vi "ALTS-2015 Display Sensor ID.vi"(8 "error in (no error)":errorcluster) -> (0 "error out":errorcluster)   [LabVIEW 2013]
doc: "Copyright © 2005, Soliton Technologies.\nAll rights reserved."
uses:
  Controls/ALTS-2015 Station Cluster.ctl
  Controls/ALTS-2015 LV2GBL Options.ctl
  Controls/ALTS-2015 LV2GBL Station Info Options.ctl
panel:
  in  "Station Enum":T1
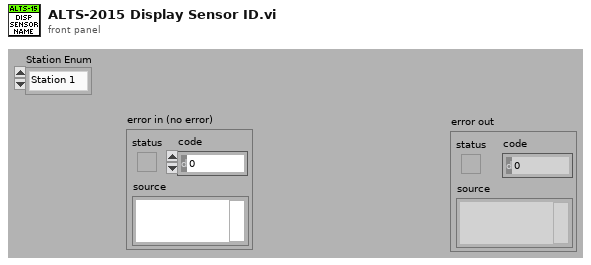
[diagram p1: front panel]
types:
  T1 = typedef "ALTS-2015 Station Cluster.ctl" = enum16{"Station 1", "Station 2", "Station 3", "Station 4"}
  T2 = typedef "ALTS-2015 LV2GBL Station Info Options.ctl" = enum16{"Init", "Read", "Read All", "Write Sensor ID", "Write  Work Order", "Write Serial Number", "Write Test Data", "Write Station Status", "Write Station Occupancy", "Write Station Test Type", "Write Rerun", "Clear All", "Clear Test Result"}
  T3 = typedef "ALTS-2015 LV2GBL Options.ctl" = enum16{"Read all", "Write all"}
  T4 = typedef "ALTS-2015 INI Configuration Cluster.ctl" = cluster{"Application":cluster{"Rerun Count":i32, "Workorder No":string}, "Station Details":cluster{"Sensor Name 1":string, "Sensor Name 2":string, "Sensor Name 3":string, "Sensor Name 4":string, "Station1 Enable":bool, "Station2 Enable":bool, "Station3 Enable":bool, "Station4 Enable":bool}, "Database":cluster{"Database Connection Link":path, "Result Procedure":string, "User":string, "Password":string, "Prompt":bool, "Station 1 LT Result DB DSN Path":path, "Station 2 LT Result DB DSN Path":path, "Station 3 LT Result DB DSN Path":path, "Station 4 LT Result DB DSN Path":path, "AirLeakTestResult Procedure":string, "Serial Details Procedure":string}, "Simulation":cluster{"Simulate DAQ Hardware":bool, "Simulate Result DB Write":bool, "Simulate Scanner":bool, "Simulate OPC":bool, "Simulate Serial Details DB":bool, "Simulate Result DB":bool, "Simulate Scanner DB Path":path, "Simulate Serial Details DB Path":path, "Simulate Result DB Path":path}, "Barcode Scanner1":cluster{"Scanner IP":string, "Scanner Port":u16, "#Bytes to Read":i32}, "Barcode Scanner2":cluster{"Enabled?":bool, "Scanner IP":string, "Scanner Port":u16, "#Bytes to Read":i32}}
  T5 = typedef "ALTS-2015 Station Details.ctl" = cluster{"Station Number":string, "Work Order Number":string, "Sensor Name":string, "Pressure (PSI)":string, "Flow (SCCM)":string, "Test Time ":string, "Test Result":string, "Serial Number":string, "Station Status":T6, "Station Occupied?":bool, "Rerun Count":i32, "Test Type":i32}
  T6 = typedef "ALTS-2015 Status Ring Indicator.ctl" = u16
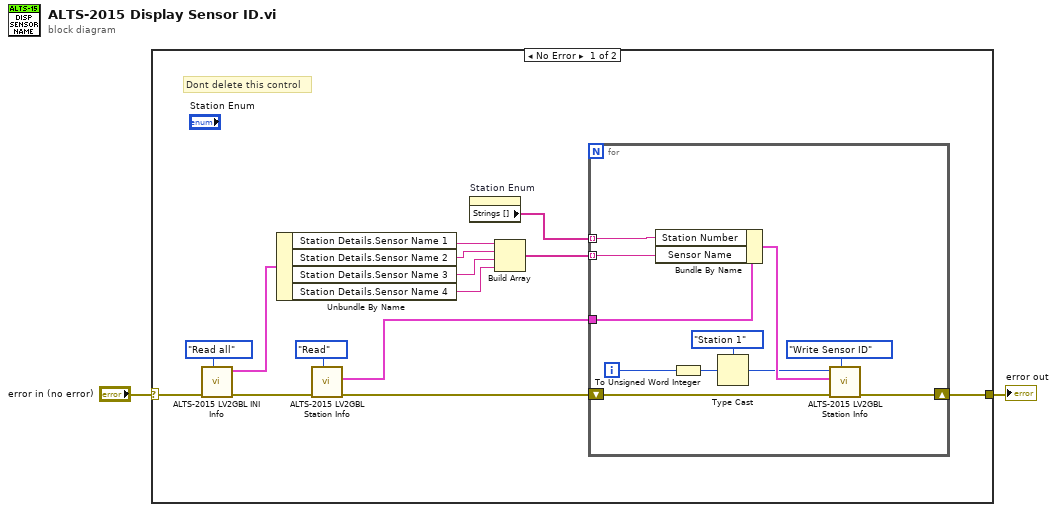
[diagram p0: block diagram]
diagram:
  n1 = case shown="No Error" "error in (no error)" {
    selector: "error in (no error)" -> [w8 w28]
    tunnel: [w6 w28] -> w1
    frame No Error {
      # "Dont delete this control"
      n2 = call "ALTS-2015 LV2GBL INI Info.vi"("Options"=ALTS-2015_LV2GBL_Options."Read all", "error in"=w8) -> ("error out"=w10:errorcluster, "Configuration Cluster Out"=w16:T4)  [unwired: 8 in]
      n3 = Unbundle By Name(w16) -> ("Station Details.Sensor Name 1"=w15:string, "Station Details.Sensor Name 2"=w14:string, "Station Details.Sensor Name 3"=w13:string, "Station Details.Sensor Name 4"=w12:string)
      n4 = call "ALTS-2015 LV2GBL Station Info.vi"("Options"=ALTS-2015_LV2GBL_Station_Info_Options."Read", "error in"=w10) -> ("error out"=w5:errorcluster, "Station Details"=w7:T5)  [unwired: 7 in, 1 out]
      n5 = property on="Station Enum" class="Enum (strict)"() -> ("Strings []"=w9:string[])  [unwired: 2 in, 2 out]
      n6 = Build Array(w15, w14, w13, w12) -> (w11:string[])
      n7 = for {
        tunnel: w11 -> [w26] mode=indexing
        tunnel: w7 -> [w27]
        tunnel: w9 -> [w25] mode=indexing
        shift-right: [w23] -> w6
        shift-left: w5 -> [w22]
        i -> [w24]
        n8 = Bundle By Name(cluster=w27, "Station Number"=w25, "Sensor Name"=w26) -> (w21:T5)
        n9 = To Unsigned Word Integer(number=w24) -> (unsigned 16bit integer=w19:u16)
        n10 = Type Cast(type=ALTS-2015_Station_Cluster."Station 1" ("Station Cluster"), x=w19) -> (*(type *) &x=w20:T1)
        n11 = call "ALTS-2015 LV2GBL Station Info.vi"("Options"=ALTS-2015_LV2GBL_Station_Info_Options."Write Sensor ID", "error in"=w22, "Station"=w21, "Station Cluster"=w20) -> ("error out"=w23:errorcluster)  [unwired: 5 in, 2 out]
      }
    }
    frame Error {
    }
  }
  "error out" <- w1
